vi "Count.vi"(8 "error in (no error)":errorcluster, 11 "BufferedArray in":refnum<class "BufferedArray.lvclass">) -> (0 "error out":errorcluster, 2 "Number of Items":i32, 3 "BufferedArray out":refnum<class "BufferedArray.lvclass">)   [LabVIEW 2013, in "LapDog.Collections.v_.Lists.Implementations.lvlib" / "BufferedArray.lvclass"]
uses:
  BufferedArray.lvclass
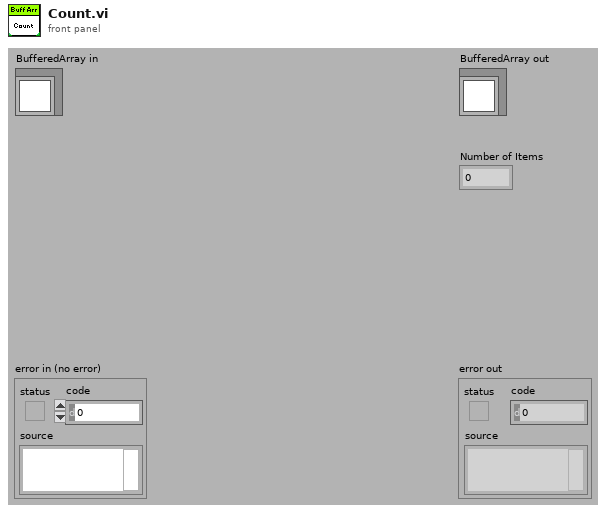
[diagram p1: front panel]
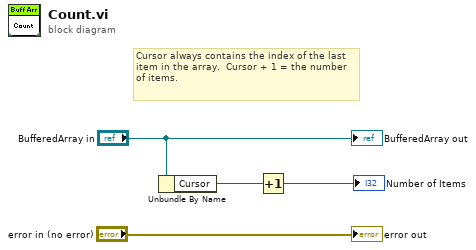
[diagram p0: block diagram]
diagram:
  # "Cursor always contains the index of the last item in the array.  Cursor + 1 = the number of items."
  n1 = Unbundle By Name("BufferedArray in") -> ("Cursor"=w2:i32)
  n2 = Increment(x=w2) -> (x+1=→"Number of Items":i32)
  "error out" <- "error in (no error)"
  "BufferedArray out" <- "BufferedArray in"
